vi "sv_Convert Value to String (Function Type).vi"(7 "function type":T1 caption="function data type") -> (8 "String":string)   [LabVIEW 2017, in "SoundVib_UFF58.lvlib"]
uses:
  <vilib>/addons/Sound and Vibration/svt_UFF58/SoundVib_UFF58.lvlib
  <vilib>/addons/Sound and Vibration/svt_UFF58/subVIs/sv_FunctionType.ctl
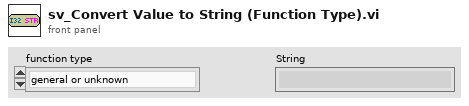
[diagram p1: front panel]
types:
  T1 = typedef "SoundVib_UFF58.lvlib/sv_FunctionType.ctl" = enum16{"general or unknown", "time response", "auto spectrum", "cross spectrum", "frequency response function", "transmissibility", "coherence", "auto correlation", "cross correlation", "power spectral density (PSD)", "energy spectral density (ESD)", "probability density function", "spectrum", "cumulative frequency distribution", "peaks valley", "stress/cycles", "strain/cycles", "orbit", "mode indicator function", "force pattern", "partial power", "partial coherence", "eigenvalue", "eigenvector", "shock response spectrum", "finite impulse response filter", "multiple coherence", "order function", "phase compensation"}
  T2 = typedef "SoundVib_UFF58.lvlib/sv_FunctionType Array.ctl" = string[]
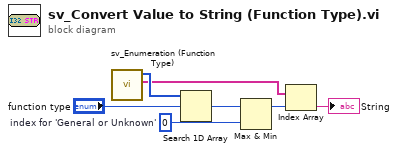
[diagram p0: block diagram]
diagram:
  w2 = 0  # index for 'General or Unknown'
  n1 = call <vilib>:"sv_Enumeration (Function Type).vi"() -> ("function type strings"=w3:T2, "function type values"=w6:T1[])  [unwired: 10 in]
  n2 = Search 1D Array(1D array=w6, element="function type") -> (index of element=w4:i32)  [unwired: 1 in]
  n3 = Max & Min(x=w4, y=w2) -> (max(x,y)=w1:i32)  [unwired: 1 out]
  n4 = Index Array(array=w3, index=w1) -> (element=→"String":string)
